vi "dfd_FXP Overflow (scaler).vi"(4 "quantization settings":T1={"source"=6, "wl"=1, "iwl"=1, "overflow mode"=enum."Saturation", "rounding mode"=enum."Nearest", "signed?"=TRUE} {"source" items=["Coef a/k"=0, "Coef b/v"=7, "Input"=1, "Output"=2, "Multiplicand"=3, "Product"=4, "Sum"=5, "Delay"=6, "Gain"=8]}, 8 "value in":dbl format="%.2f") -> (1 "# underflow":i32, 2 "# overflow":i32, 3 "value out":dbl format="%.2f")   [LabVIEW 2017, in "NI_DigFilter_FXP.lvlib"]
uses:
  <vilib>/addons/Digital Filter Design/NI_DigFilter_FXP.lvlib
  <vilib>/addons/Digital Filter Design/_Objects.llb/dfd_Internal Quantization Settings.ctl
  <vilib>/addons/Digital Filter Design/_Objects.llb/dfd_Internal Quantization Srcs.ctl
  <vilib>/addons/Digital Filter Design/NI_DigFilterLicensed.lvlib
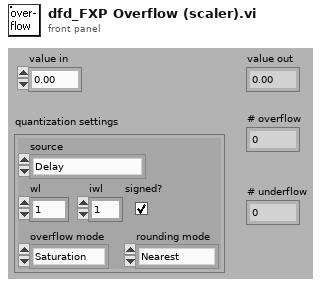
[diagram p1: front panel]
types:
  T1 = typedef "NI_DigFilterLicensed.lvlib/dfd_Internal Quantization Settings.ctl" = cluster{"source":T2, "wl":i16, "iwl":i16, "overflow mode":enum16{"Saturation", "Wrap"}, "rounding mode":enum16{"Nearest", "Truncation"}, "signed?":bool}
  T2 = typedef "NI_DigFilterLicensed.lvlib/dfd_Internal Quantization Srcs.ctl" = u16
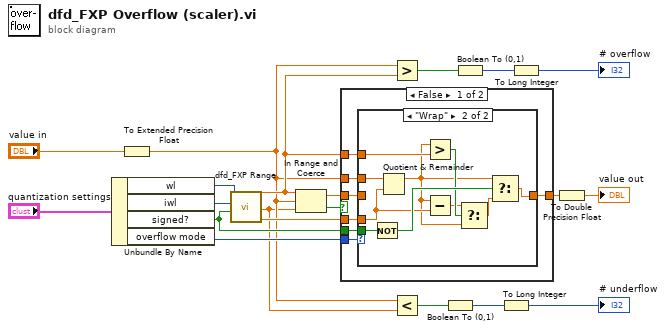
[diagram p0: block diagram]
diagram:
  n1 = Unbundle By Name("quantization settings") -> ("wl"=w2:i16, "iwl"=w1:i16, "signed?"=w16:bool, "overflow mode"=w18:enum16{"Saturation", "Wrap"})
  n2 = To Extended Precision Float(1:"value in") -> (0:w7:ext)
  n3 = call <vilib>:"dfd_FXP Range.vi"("signed?"=w16, "iwl"=w1, "wl"=w2) -> ("full range"=w17:ext, "low"=w6:ext, "high"=w11:ext)  [unwired: 6 out]
  n4 = In Range and Coerce(upper limit=w11, x=w7, lower limit=w6) -> (coerced(x)=w19:ext, In Range?=w20:bool)
  n5 = case shown="False" w20 {
    tunnel: [w25 w39] -> w13
    tunnel: w19 -> [w26 w39]
    tunnel: w18 -> [w27 _]
    tunnel: w17 -> [w24 _]
    tunnel: w7 -> [w23 _]
    tunnel: w16 -> [w22 _]
    tunnel: w11 -> [w21 _]
    frame False {
      n6 = case shown="\"Wrap\"" w27 {
        tunnel: [w28 w37] -> w25
        tunnel: w26 -> [w28 _]
        tunnel: w24 -> [_ w31]
        tunnel: w23 -> [_ w38]
        tunnel: w22 -> [_ w36]
        tunnel: w21 -> [_ w34]
        frame "Saturation", Default {
        }
        frame "Wrap" {
          n7 = Not(x=w36) -> (.not. x?=w35:bool)
          n8 = Quotient & Remainder(x=w38, y=w31) -> (x-y*floor(x/y)=w30:ext)  [unwired: 1 out]
          n9 = Greater?(x=w30, y=w34) -> (0:w33:bool)
          n10 = Subtract(x=w30, y=w31) -> (x-y=w32:ext)
          n11 = Select(t=w32, s=w33, f=w30) -> (s? t:f=w29:ext)
          n12 = Select(t=w30, s=w35, f=w29) -> (s? t:f=w37:ext)
        }
      }
    }
    frame True {
    }
  }
  n13 = Greater?(x=w7, y=w11) -> (0:w9:bool)
  n14 = Less?(x=w7, y=w6) -> (x < y?=w3:bool)
  n15 = Boolean To (0,1)(Boolean=w3) -> (0, 1=w4:i16)
  n16 = Boolean To (0,1)(Boolean=w9) -> (0, 1=w10:i16)
  n17 = To Long Integer(number=w4) -> (32bit integer=→"# underflow":i32)
  n18 = To Long Integer(number=w10) -> (32bit integer=→"# overflow":i32)
  n19 = To Double Precision Float(number=w13) -> (double precision float=→"value out":dbl)
